vi "CalibratePosition.vi"(3 "error in (no error)":errorcluster, 4 "Current Wavelength":u16, 5 "VISA resource name":refnum<visa-resource-name>) -> (0 "error out":errorcluster, 1 "Command not accepted":bool, 2 "VISA resource name out":refnum<visa-resource-name>)   [LabVIEW 2017]
uses:
  Spectral Products CM110.lvlib
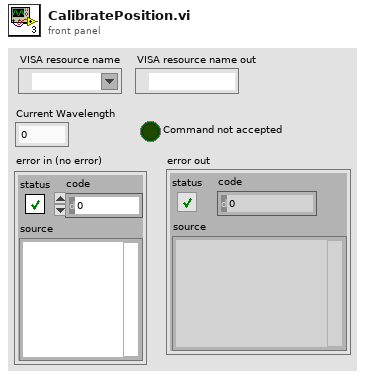
[diagram p1: front panel]
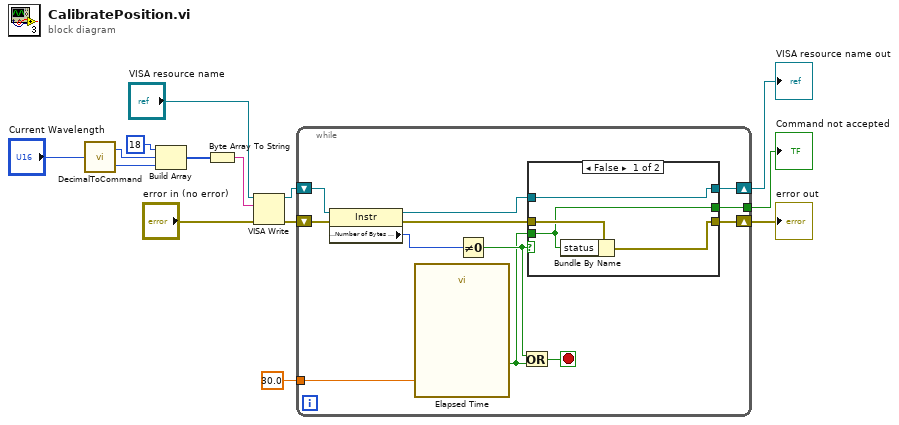
[diagram p0: block diagram]
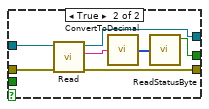
[diagram p2: hidden frame]
diagram:
  n1 = call "DecimalToCommand.vi"("Decimal"="Current Wavelength") -> ("HiByte"=w10:u8, "LoByte"=w9:u8)  [unwired: 4 in]
  n2 = Build Array(u8 18, w10, w9) -> (w8:u8[])
  n3 = Byte Array To String(unsigned byte array=w8) -> (string=w7:string)
  n4 = VISA Write(VISA resource name="VISA resource name", write buffer=w7, error in (no error)="error in (no error)") -> (VISA resource name out=w2:refnum<visa-resource-name>, error out=w1:errorcluster)  [unwired: 1 out]
  n5 = while {
    tunnel: 30.0 ("Time Target (s)") -> [w23]
    shift-right: [w19] -> w4
    shift-left: w2 -> [w18]
    shift-right: [w20] -> w5
    shift-left: w1 -> [w17]
    tunnel: [w15] -> w3
    stop <- w21 stop-if-true
    n6 = property class="Instr"(reference=w18, error in=w17) -> (reference out=w25:refnum<visa-resource-name>, error out=w24:errorcluster, "Serial Settings:Number of Bytes at Serial Port"=w26:u32)
    n7 = call "Elapsed Time"("Time Target (s)"=w23) -> ("Time has Elapsed"=w16:bool)  [unwired: 11 in, 7 out]
    n8 = Not Equal To 0?(x=w26) -> (x != 0?=w22:bool)
    n9 = Or(x=w22, y=w16) -> (x .or. y?=w21:bool)
    n10 = case shown="False" w22 {
      tunnel: w25 -> [w30 w37]
      tunnel: w24 -> [w29 w36]
      tunnel: [w28 w33] -> w20
      tunnel: [w30 w32] -> w19
      tunnel: w16 -> [w27 _]
      tunnel: [w27 w31] -> w15
      frame False {
        n11 = Bundle By Name(cluster=w29, "status"=w27) -> (w28:errorcluster)
      }
      frame True {
        n12 = call "Read.vi"("error in (no error)"=w36, "VISA Refnum in"=w37) -> ("error out"=w33:errorcluster, "read buffer"=w34:string, "VISA Refnum out"=w32:refnum<visa-resource-name>)  [unwired: 6 in, 1 out]
        n13 = call "ConvertToDecimal.vi"("read buffer"=w34) -> ("unsigned byte array"=w35:u8[])
        n14 = call "ReadStatusByte.vi"("unsigned byte array"=w35) -> ("Command not accepted"=w31:bool)  [unwired: 4 in, 5 out]
      }
    }
  }
  "VISA resource name out" <- w4
  "error out" <- w5
  "Command not accepted" <- w3
